vi "Do.vi"(8 "error in (no error)":errorcluster, 10 "Actor in":refnum<class "Actor.lvclass">, 11 "WebSocket Connection Handler Msg":refnum<class "WebSocket Connection Handler Msg.lvclass">) -> (0 "error out":errorcluster, 2 "Actor out":refnum<class "Actor.lvclass">)   [LabVIEW 2016, in "WebSocket Actors.lvlib" / "WebSocket Connection Handler Msg.lvclass"]
doc: "(<B>Filename</B>: Actor Framework.lvlib:Message.lvclass:Do.vi)\n\nDefines what a message does when it is received by an actor. Generally, a message instructs an actor to invoke one of its methods. By default, this method does nothing. A child class must override it to define behavior. Create a child class by using the Actor Framework Message Maker dialog box."
uses:
  WebSocket Connection Handler Msg.lvclass
  <vilib>/ActorFramework/Actor/Actor.lvclass
  WebSocket Connection Handler Msg.lvclass/WebSocket Connection Handler Msg.ctl
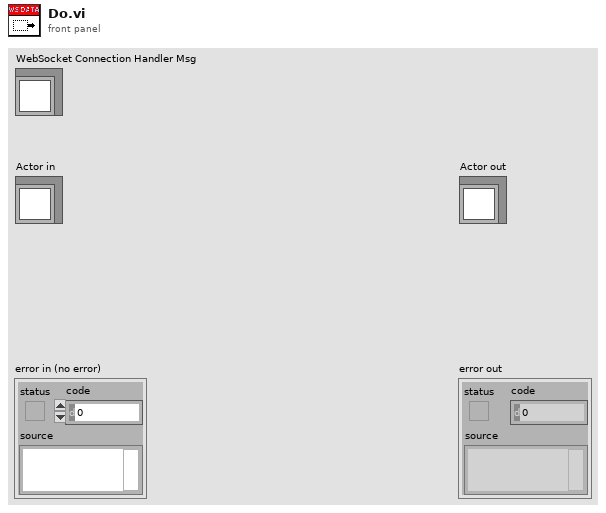
[diagram p1: front panel]
types:
  T1 = typedef "WebSocket Actors.lvlib/WebSocket Connection Handler Msg.lvclass/Connection Event.ctl" = enum16{"On Connect", "On Message", "On Close", "On Drop"}
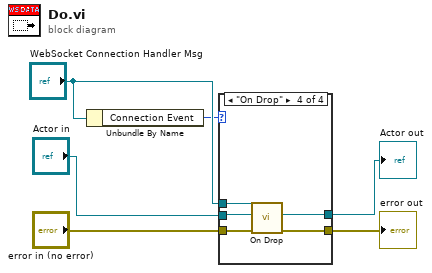
[diagram p0: block diagram]
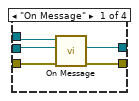
[diagram p2: hidden frame]
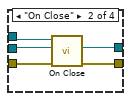
[diagram p3: hidden frame]
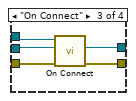
[diagram p4: hidden frame]
diagram:
  n1 = Unbundle By Name("WebSocket Connection Handler Msg") -> ("Connection Event"=w1:T1)
  n2 = case shown="\"On Drop\"" w1 {
    tunnel: [w11 w16 w21 w25] -> w6
    tunnel: [w7 w12 w17 w24] -> w5
    tunnel: "error in (no error)" -> [w10 w15 w20 w26]
    tunnel: "Actor in" -> [w9 w14 w19 w23]
    tunnel: "WebSocket Connection Handler Msg" -> [w8 w13 w18 w22]
    frame "On Message" {
      n3 = call-dynamic "On Message.vi"("error in (no error)"=w10, "Actor in"=w9, "WebSocket Connection Handler Msg in"=w8) -> ("error out"=w11:errorcluster, "Actor out"=w7:refnum<class "Actor.lvclass">)  [unwired: 6 in, 1 out]
    }
    frame "On Close" {
      n4 = call-dynamic "On Close.vi"("error in (no error)"=w15, "Actor in"=w14, "WebSocket Connection Handler Msg in"=w13) -> ("error out"=w16:errorcluster, "Actor out"=w12:refnum<class "Actor.lvclass">)  [unwired: 6 in, 1 out]
    }
    frame "On Connect" {
      n5 = call-dynamic "On Connect.vi"("error in (no error)"=w20, "Actor in"=w19, "WebSocket Connection Handler Msg in"=w18) -> ("error out"=w21:errorcluster, "Actor out"=w17:refnum<class "Actor.lvclass">)  [unwired: 6 in, 1 out]
    }
    frame "On Drop" {
      n6 = call-dynamic "On Drop.vi"("error in (no error)"=w26, "Actor in"=w23, "WebSocket Connection Handler Msg in"=w22) -> ("error out"=w25:errorcluster, "Actor out"=w24:refnum<class "Actor.lvclass">)  [unwired: 6 in, 1 out]
    }
  }
  "error out" <- w6
  "Actor out" <- w5
